vi "Disconnect All.vi"(8 "error in (no error)":errorcluster, 11 "SLSC Switch Consumer in":refnum<class "SLSC Switch Consumer.lvclass">) -> (0 "error out":errorcluster, 3 "SLSC Switch Consumer out":refnum<class "SLSC Switch Consumer.lvclass">)   [LabVIEW 2017, in "SLSC Switch Consumer.lvclass"]
uses:
  SLSC Switch Consumer.lvclass
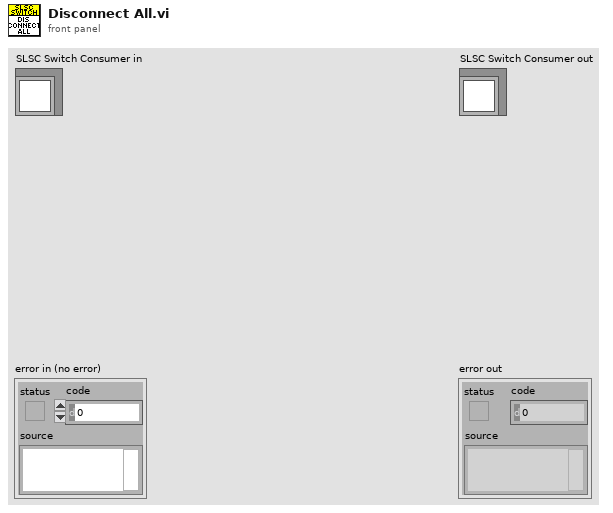
[diagram p1: front panel]
types:
  T1 = typedef "nislscslSession.ctl" = refnum<k20>
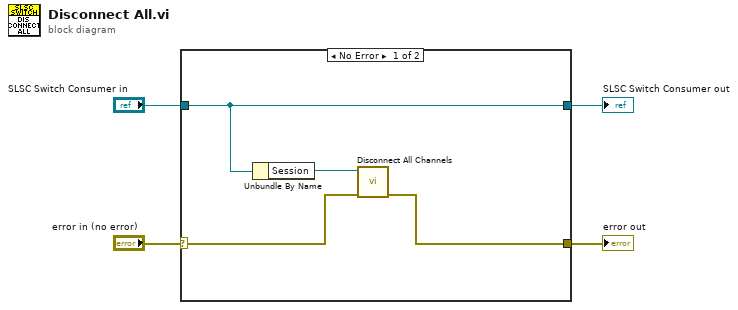
[diagram p0: block diagram]
diagram:
  n1 = case shown="No Error" "error in (no error)" {
    selector: "error in (no error)" -> [w6 w10]
    tunnel: [w5 w10] -> w1
    tunnel: [w8 w9] -> w3
    tunnel: "SLSC Switch Consumer in" -> [w8 w9]
    frame No Error {
      n2 = Unbundle By Name(w8) -> ("Session"=w7:T1)
      n3 = call <vilib>:"Disconnect All Channels.vi"("error in (no error)"=w6, "session in"=w7) -> ("error out"=w5:errorcluster)  [unwired: 8 in, 1 out]
    }
    frame Error {
    }
  }
  "error out" <- w1
  "SLSC Switch Consumer out" <- w3
